vi "Intake And Elevator Mode Select.vi"(10 "Key Pressed?":bool) -> ()   [LabVIEW 2017]
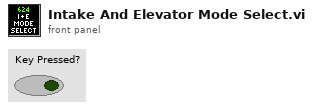
[diagram p1: front panel]
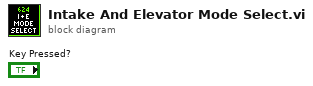
[diagram p0: block diagram]
diagram:
